vi "Set BME G05.vi"(7 "Settings":T1={"T Delay (µs)"=0.0, "T Set Back"=0.0, "T Triggers"=1, "T Active"=TRUE, "T Polarity"=TRUE, "T Term"=TRUE, "T Drive"=FALSE, "A Delay (µs)"=0.0, "A Set Back"=0.0, "A Triggers"=1, "A Active"=TRUE, "A Polarity"=TRUE, "A Term"=TRUE, "A Drive"=FALSE, "B Delay (µs)"=0.0, "B Set Back"=0.0, "B Triggers"=1, "B Active"=TRUE, "B Polarity"=TRUE, "B Term"=TRUE, "B Drive"=FALSE, "Gate A*B"=FALSE, "Output\nLevel"=1, "Trigger\nTerminate"=TRUE, "Clock\nEnable"=TRUE, "Internal\nClock (µs)"=0.0125, "Trigger\nLevel"=0.2, "Stop\nTrigger"=1, "Ocillator\nDivide By"=1, "Clock Source"=3, "Gate Divider"=1, "Positive\nGate"=FALSE, "Trigger\nSource"=FALSE, "Internal\nArming"=FALSE, "Software\nTrigger"=FALSE, "Trigger\nSlope"=TRUE, "Stop on\nPreset"=FALSE, "Trigger\nOperation"=TRUE, "Trigger\nEnable"=TRUE} {"B Set Back" min=0.0 format="%.3f"; "A Set Back" min=0.0 format="%.3f"; "T Set Back" min=0.0 format="%.3f"; "Clock Source" items=["Internal Oscillator"=1, "External Trigger"=2, "Trigger & Oscillator"=3, "Master Slave Bus"=4]; "Trigger\nLevel" min=0.0 format="%.3f"; "Output\nLevel" items=["TTL"=1, "NIM"=2, "ECL"=3]; "Internal\nClock (µs)" min=0.0 format="%.4f"; "B Delay (µs)" min=0.0 format="%.3f"; "A Delay (µs)" min=0.0 format="%.3f"; "T Delay (µs)" min=0.0 format="%.3f"}, 8 "error in (no error)":errorcluster, 10 "External Prescaler":u16=3, 11 "DG Number":i32) -> (0 "error out":errorcluster)   [LabVIEW 2009]
doc: "long Set_BME_G05(double FireFirst_T0, unsigned long OutputModulo_T0, BOOL Active_T0, BOOL Positive_T0, BOOL Terminate_T0, BOOL HighDrive_T0, double FireFirst_A, unsigned long OutputModulo_A, BOOL Active_A, BOOL Positive_A, BOOL Terminate_A, BOOL HighDrive_A, double FireFirst_B, unsigned long OutputModulo_B, BOOL Active_B, BOOL Positive_B, BOOL Terminate_B, BOOL HighDrive_B, BOOL Gate_AB, unsigned long OutputLevel, BOOL TriggerTerminate, BOOL ClockEnable, double InternalClock, double TriggerLevel, unsigned long PresetValue, unsigned long DivideBy, unsigned long ClockSource, unsigned long GateDivider, BOOL PositiveGate, BOOL InternalTrigger, BOOL InternalArm, BOOL SoftwareTrigger, BOOL RisingEdge, BOOL StopOnPreset, BOOL ResetWhenDone, BOOL TriggerEnable, long DG_Number);"
uses:
  Settings.ctl
  BME DLL/DelayGenerator.dll
panel:
  # "NOTICE -- YOU MUST LEAVE THIS NOTICE IN PLACE.  PER THE TERMS OF THE LICENSE BELOW, YOU MAY SUBLICENSE THIS SOFTWARE \nIN ANY WAY THAT DOES NOT CONFLICT WITH THIS LICENSE.\n\n### BSD License (http://www.opensource.org/licenses/bsd-license.php) Begin ###\n \nCopyright (c) 2011, Applied Energetics, http://www.appliedenergetics.com,\n                               Richard Schwerdtfeger, <rschwerdtfeger@appliedenergetics.com>\n\nAll rights reserved.\n\nRedistribution and use in source and binary forms, with or without modification, are permitted provided that the \nfollowing conditions are met:\n\n    * Redistributions of source code must retain the above copyright notice, this list of conditions and the following disclaimer.\n    * Redistributions in binary form must reproduce the above copyright notice, this list of conditions and the following disclaimer \n       in the documentation and/or other materials provided with the distribution.\n    * Neither the name of Richard Schwerdtfeger, Applied Energetics, Inc., nor the names of its contributors may be used to \n       endorse or promote products derived from this software without specific prior written permission.\n\nTHIS SOFTWARE IS PROVIDED BY THE COPYRIGHT HOLDERS AND CONTRIBUTORS \"AS IS\" AND ANY EXPRESS OR IMPLIED WARRANTIES, \nINCLUDING, BUT NOT LIMITED TO, THE IMPLIED WARRANTIES OF MERCHANTABILITY AND FITNESS FOR A PARTICULAR PURPOSE ARE \nDISCLAIMED. IN NO EVENT SHALL THE COPYRIGHT OWNER OR CONTRIBUTORS BE LIABLE FOR ANY DIRECT, INDIRECT, INCIDENTAL,\n SPECIAL, EXEMPLARY, OR CONSEQUENTIAL DAMAGES (INCLUDING, BUT NOT LIMITED TO, PROCUREMENT OF SUBSTITUTE GOODS OR \nSERVICES; LOSS OF USE, DATA, OR PROFITS; OR BUSINESS INTERRUPTION) HOWEVER CAUSED AND ON ANY THEORY OF LIABILITY, \nWHETHER IN CONTRACT, STRICT LIABILITY, OR TORT (INCLUDING NEGLIGENCE OR OTHERWISE) ARISING IN ANY WAY OUT OF THE USE \nOF THIS SOFTWARE, EVEN IF ADVISED OF THE POSSIBILITY OF SUCH DAMAGE.\n\n### BSD License End ###"
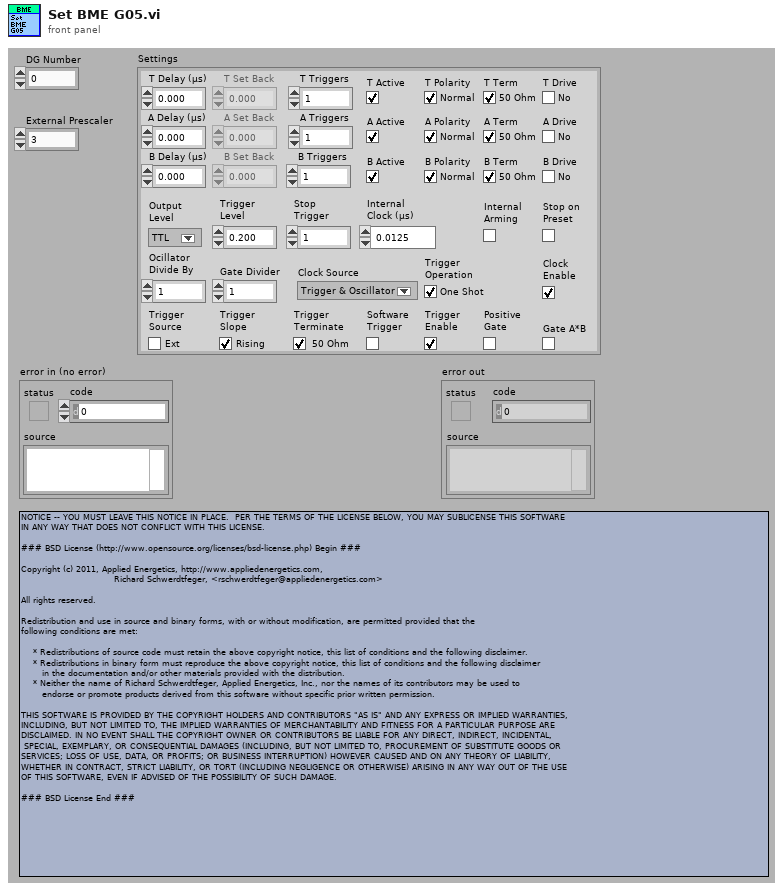
[diagram p1: front panel]
types:
  T1 = typedef "Settings.ctl" = cluster{"T Delay (µs)":dbl, "T Set Back":dbl, "T Triggers":u16, "T Active":bool, "T Polarity":bool, "T Term":bool, "T Drive":bool, "A Delay (µs)":dbl, "A Set Back":dbl, "A Triggers":u16, "A Active":bool, "A Polarity":bool, "A Term":bool, "A Drive":bool, "B Delay (µs)":dbl, "B Set Back":dbl, "B Triggers":u16, "B Active":bool, "B Polarity":bool, "B Term":bool, "B Drive":bool, "Gate A*B":bool, "Output\nLevel":u32, "Trigger\nTerminate":bool, "Clock\nEnable":bool, "Internal\nClock (µs)":dbl, "Trigger\nLevel":dbl, "Stop\nTrigger":u32, "Ocillator\nDivide By":u16, "Clock Source":u32, "Gate Divider":u32, "Positive\nGate":bool, "Trigger\nSource":bool, "Internal\nArming":bool, "Software\nTrigger":bool, "Trigger\nSlope":bool, "Stop on\nPreset":bool, "Trigger\nOperation":bool, "Trigger\nEnable":bool}
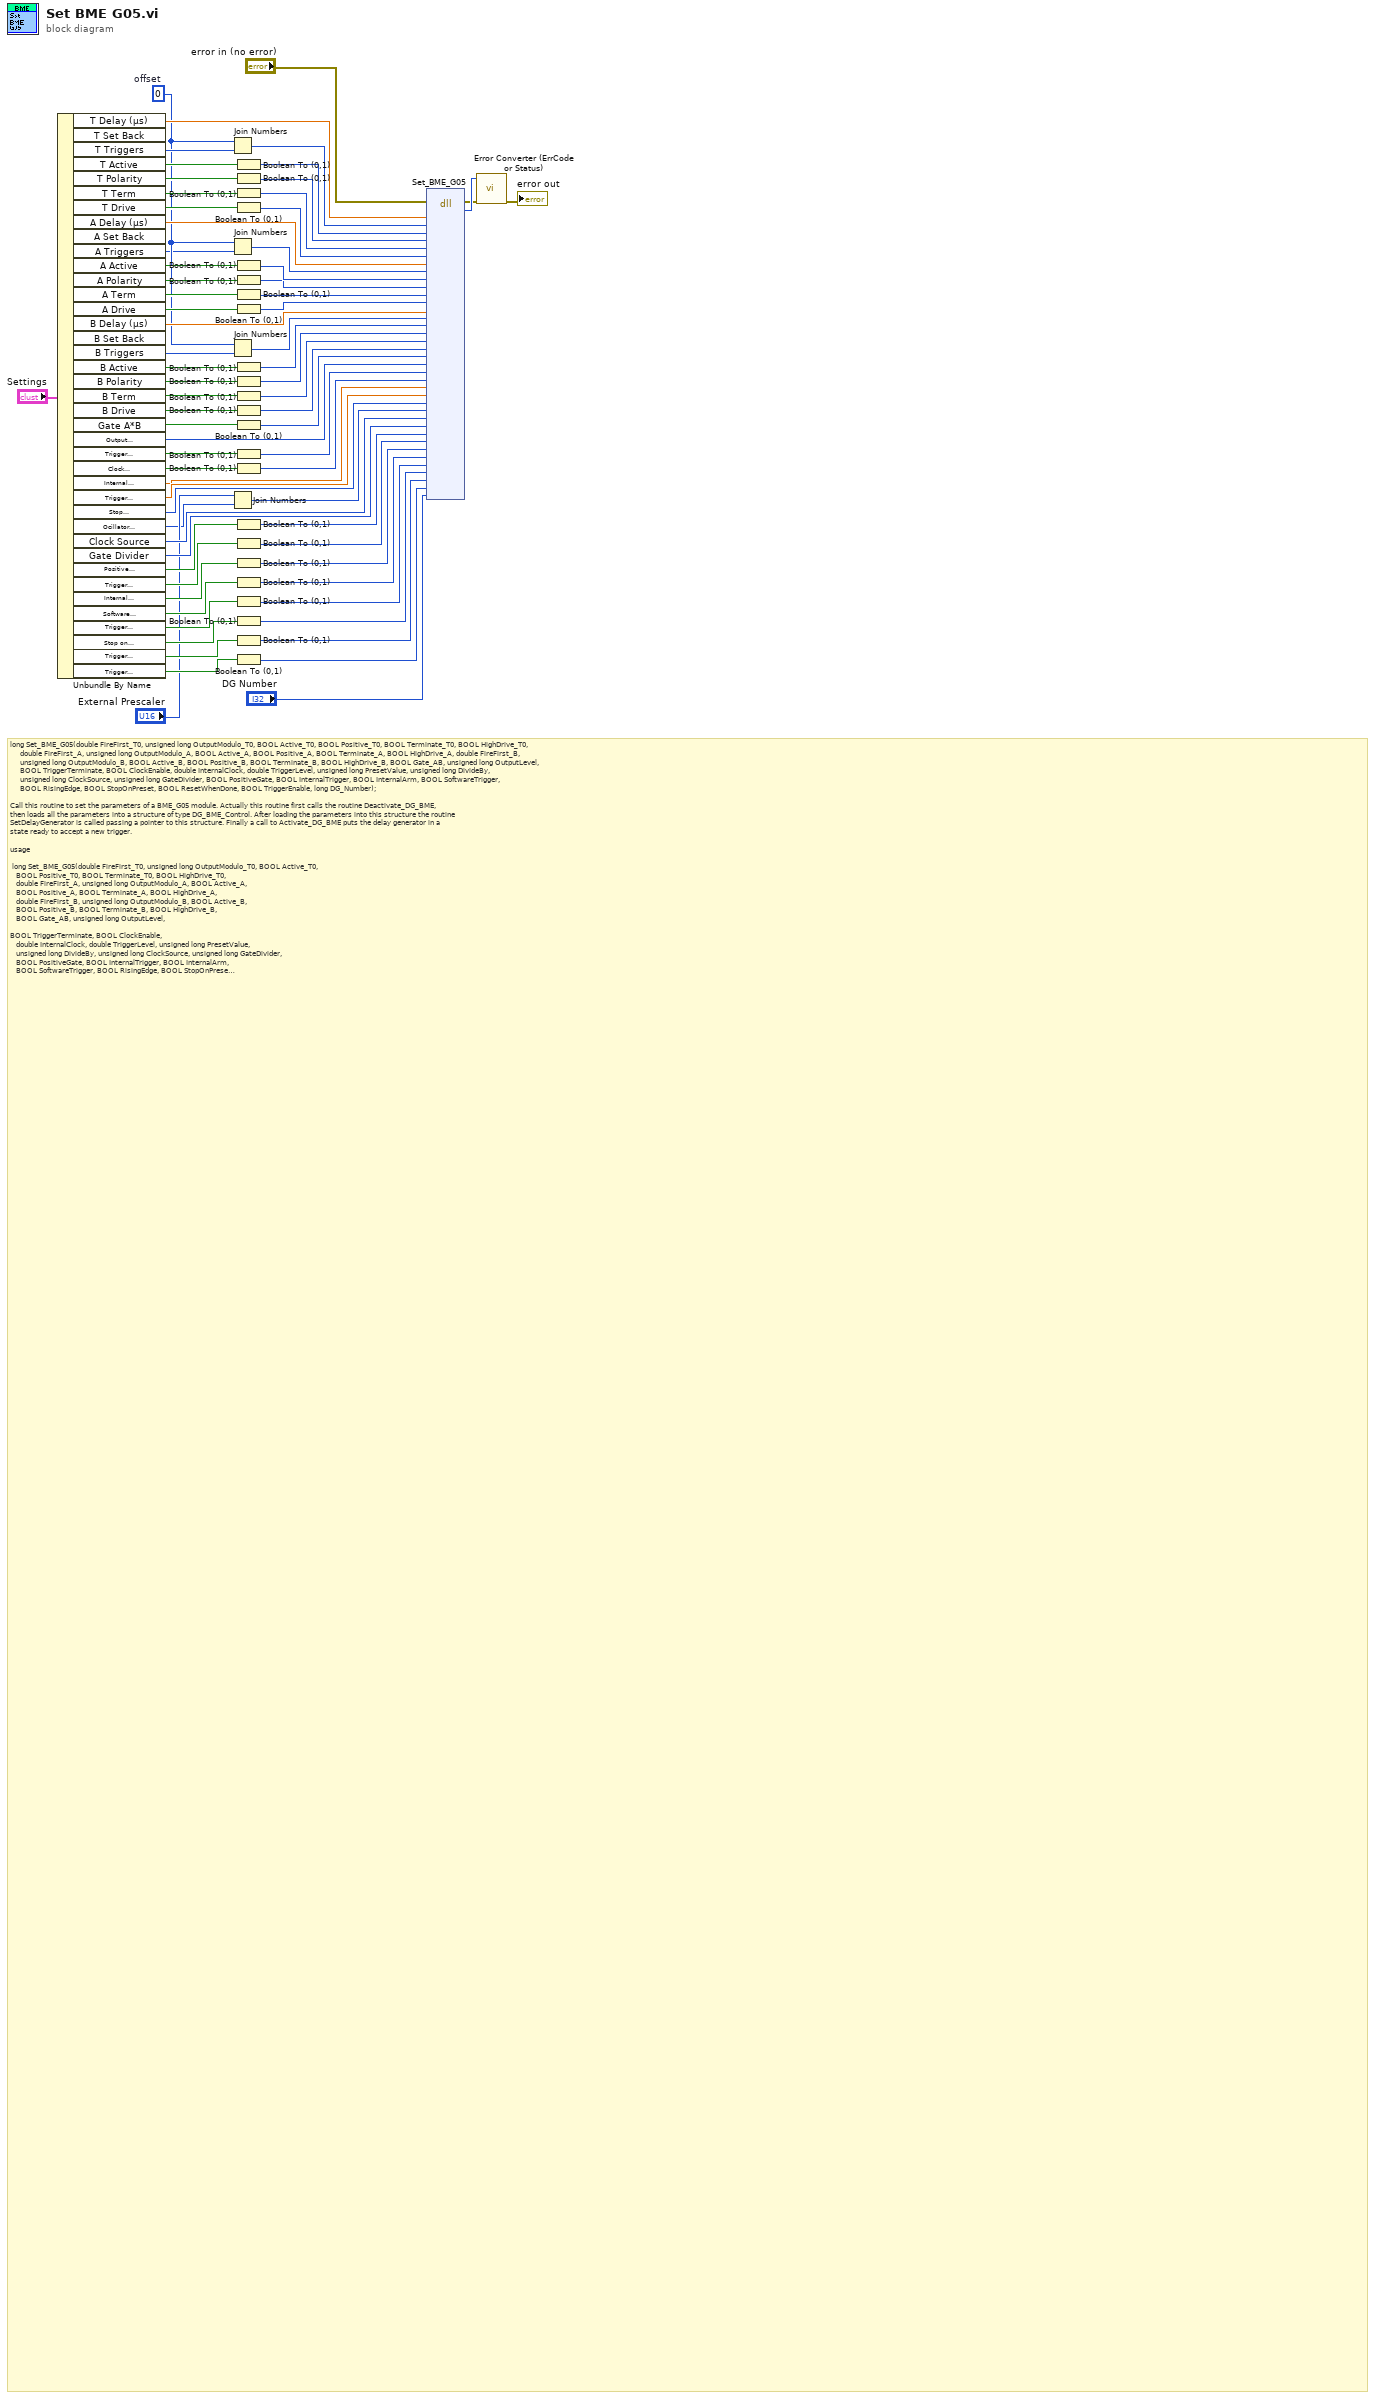
[diagram p0: block diagram]
diagram:
  w5 = u16 0  # offset
  # "long Set_BME_G05(double FireFirst_T0, unsigned long OutputModulo_T0, BOOL Active_T0, BOOL Positive_T0, BOOL Terminate_T0, BOOL HighDrive_T0, \n     double FireFirst_A, unsigned long OutputModulo_A, BOOL Active_A, BOOL Positive_A, BOOL Terminate_A, BOOL HighDrive_A, double FireFirst_B, \n     unsigned long OutputModulo_B, BOOL Active_B, BOOL Positive_B, BOOL Terminate_B, BOOL HighDrive_B, BOOL Gate_AB, unsigned long OutputLevel, \n     BOOL TriggerTerminate, BOOL ClockEnable, double InternalClock, double TriggerLevel, unsigned long PresetValue, unsigned long DivideBy, \n     unsigned long ClockSource, unsigned long GateDivider, BOOL PositiveGate, BOOL InternalTrigger, BOOL InternalArm, BOOL SoftwareTrigger, \n     BOOL RisingEdge, BOOL StopOnPreset, BOOL ResetWhenDone, BOOL TriggerEnable, long DG_Number);\n\nCall this routine to set the parameters of a BME_G05 module. Actually this routine first calls the routine Deactivate_DG_BME, \nthen loads all the parameters into a structure of type DG_BME_Control. After loading the parameters into this structure the routine \nSetDelayGenerator is called passing a pointer to this structure. Finally a call to Activate_DG_BME puts the delay generator in a \nstate ready to accept a new trigger.\n\nusage\n\n\tlong Set_BME_G05(double FireFirst_T0, unsigned long OutputModulo_T0, BOOL Active_T0,\n\t\t\tBOOL Positive_T0, BOOL Terminate_T0, BOOL HighDrive_T0,\n\t\t\tdouble FireFirst_A, unsigned long OutputModulo_A, BOOL Active_A,\n\t\t\tBOOL Positive_A, BOOL Terminate_A, BOOL HighDrive_A,\n\t\t\tdouble FireFirst_B, unsigned long OutputModulo_B, BOOL Active_B,\n\t\t\tBOOL Positive_B, BOOL Terminate_B, BOOL HighDrive_B,\n\t\t\tBOOL Gate_AB, unsigned long OutputLevel,\n\nBOOL TriggerTerminate, BOOL ClockEnable,\n\t\t\tdouble InternalClock, double TriggerLevel, unsigned long PresetValue,\n\t\t\tunsigned long DivideBy, unsigned long ClockSource, unsigned long GateDivider,\n\t\t\tBOOL PositiveGate, BOOL InternalTrigger, BOOL InternalArm,\n\t\t\tBOOL SoftwareTrigger, BOOL RisingEdge, BOOL StopOnPreset,\n\t\t\tBOOL ResetWhenDone, BOOL TriggerEnable, long DG_Number);\n\nparameters\n\nFireFirst_T0:    time after the main trigger in µsec, when the output T0 should be set\nOutputModulo_T0:    for every number of trigger events specified in this variable, only one pulse will actually be output at the T0 connector of the delay generator. \n\t\t\tActually this variable consists of two 16-bit numbers, the lower 16 bits actually specifying the number of triggers that have to occur for one pulse to come from the output connector. \n\t\t\tFor the delay generator models BME_G05P2 and BME_SG05P1 the higher 16 bits of this variable specify the offset when starting to count the triggers until a pulse comes from the \n\t\t\toutput connector. Note that after modifying this value, it is advisable to call the routine ResetOutputModuloCounters to resynchronize the output modulo counters.\nActive_T0:    TRUE to specify an output from T0, otherwise FALSE\nPositive_T0:    TRUE to specify a positive output polarity from T0, otherwise FALSE\nTerminate_T0:    TRUE to specify an internal 50 ohm termination on output T0, otherwise FALSE\nHighDrive_T0:    TRUE to specify a high current source driving a 25 ohm output, otherwise FALSE\n\nFireFirst_A:    time after the main trigger in µsec, when the output A should be set\nOutputModulo_A:    same as OutputModulo_T0 for output A\nActive_A:    TRUE to specify an output from A, otherwise FALSE\nPositive_A:    TRUE to specify a positive output polarity from A, otherwise FALSE\nTerminate_A:    TRUE to specify an internal 50 ohm termination on output A, otherwise FALSE\nHighDrive_A:    TRUE to specify a high current source driving a 25 ohm output, otherwise FALSE\n\nFireFirst_B:    time after the main trigger in µsec, when the output B should be set\nOutputModulo_B:    same as OutputModulo_T0 for output B\nActive_B:    TRUE to specify an output from B, otherwise FALSE\nPositive_B:    TRUE to specify a positive output polarity from B, otherwise FALSE\nTerminate_B:    TRUE to specify an internal 50 ohm termination on output B, otherwise FALSE\nHighDrive_B:    TRUE to specify a high current source driving a 25 ohm output, otherwise FALSE\n\nGate_AB:    if this flag is set, outputs A and B will be combined to form a gate signal, i.e. FireFirst_A will define the time when the output signal is set, and FireFirst_B will define the\n\t\t\ttime when the output signal is reset. Note that both outputs A and B must be activated, if the gate function is to be activated.\nOutputLevel:    specifies the voltage levels on the outputs of the delay generator. The constants for this variable are defined in ‘’DG_Data.h’’. (TTL_VoltageLevel, NIM_VoltageLevel, ECL_VoltageLevel)\nTriggerTerminate:    TRUE to specify an internal 50 ohm termination on the trigger input, otherwise FALSE\nClockEnable:    this flag must be set to enable the clock circuit\nInternalClock:    period of the internal clock in µsec. The BME_SG02p3 delay generator understands this entry as the trigger inhibit time.\nTriggerLevel:    Voltage of the trigger threshold. Can be varied from -2.5V to +2.5V\nPresetValue:    the BME_G02 will disable its trigger circuit after this number of trigger signals has occurred, provided the StopOnPreset flag is set.\nDivideBy:    this variable consists of two 16-bit unsigned short values. The lower signifying the prescaler value of the internal quarz oscillator, the higher giving the prescaler value for the \n\t\t\texternal clock signal fed via the trigger input connector\nClockSource:        the source of the clock signal, can be the crystal oscillator or a signal fed to the external trigger input. (The constants for this variable, CrystalOscillator or TriggerInput, are defined in ‘’DG_Data.h’’.)\n    CrystalOscillator = 1:    internal quarz oscillator is used\n    TriggerInput = 2:         signal from external trigger/clock input connector is used\n    TriggerAndOscillator = 3:     like TriggerInput, but if this signal fails, the signal from the internal quarz oscillator will be used.\n\nGateDivider:    the external gate signal will be divided by this number.\nPositiveGate:    set this flag to TRUE, if a positive signal on the external gate input should enable the trigger circuit, otherwise FALSE. Note that the TriggerEnable flag is or’ed \n\t\t\twith the external gate signal. Only when the TriggerEnable flag is set FALSE, the trigger circuit can be enabled by the external gate signal.\nInternalTrigger:    if this flag is set the BME_G02 will be triggered by its internal clock, (provided it is jumpered as a master module).\nInternalArm:    if this flag is set the external trigger of the BME_G02 will be armed by its internal clock, (provided it is jumpered as a master module).\nSoftwareTrigger:        if this flag is set the BME_G02 will be triggered by the SoftwareTrigger_DG_BME routine, (provided it is jumpered as a master module). The flags InternalTrigger and\n\t\t\t SoftwareTrigger may not be set at the same time.\nRisingEdge:    if none of the flags InternalTrigger or SoftwareTrigger are set and this module is jumpered as master, the BME_G02 will be triggered by the rising edge of a signal applied to its external connector.\nStopOnPreset:    if this flag is set, the BME_G02 will disable its trigger circuit when the number of triggers prescribed by PresetValue has been reached. Modules slaved to a master will also stop at this point.\nResetWhenDone:    if this flag is set, all outputs from master and slave(s) will be reset to their untriggered states 2 µsec after the last delay of master and slave(s) has elapsed. This function is controlled by \n\t\t\tthe master module. If this flag is not set, all modules, master and slave(s) have to be individually reset by calling the two routines Deactivate_DG_BME and Activate_DG_BME (in that order).\nTriggerEnable:    this flag must be set to enable the trigger circuit. This signal is or'ed with the signal coming from the external gate input. Actually, the rising edge of the (divided) gate signal clocks a flip-flop \n\t\t\tallowing a trigger. After a trigger has occurred, the flip-flop is reset.\nDG_Number:    The number of the delay generator as assigned by the Initialize_DG_BME routine\n\n\nreturn value\n\n0:  success\n2:  DG_Number is out of range\n3:  the FireFirst time of an output is negative while the Active flag is TRUE.\n4:  more than one of the flags InternalTrigger, InternalArm, and SoftwareTrigger have both been set\n5:  one or more delay time(s) is specified too long\n6:  parameter ‘OutputLevel’ has been passed with illegal value. (See DG_Data.h)\n7:  parameter ‘ClockSource’ has been passed with illegal value. (See DG_Data.h)"
  n1 = Unbundle By Name("Settings") -> ("T Delay (µs)"=w44:dbl, "T Triggers"=w7:u16, "T Active"=w47:bool, "T Polarity"=w48:bool, "T Term"=w49:bool, "T Drive"=w50:bool, "A Delay (µs)"=w39:dbl, "A Triggers"=w2:u16, "A Active"=w51:bool, "A Polarity"=w52:bool, "A Term"=w53:bool, "A Drive"=w54:bool, "B Delay (µs)"=w34:dbl, "B Triggers"=w1:u16, "B Active"=w58:bool, "B Polarity"=w55:bool, "B Term"=w56:bool, "B Drive"=w57:bool, "Gate A*B"=w61:bool, "Output\nLevel"=w28:u32, "Trigger\nTerminate"=w59:bool, "Clock\nEnable"=w60:bool, "Internal\nClock (µs)"=w8:dbl, "Trigger\nLevel"=w25:dbl, "Stop\nTrigger"=w24:u32, "Ocillator\nDivide By"=w10:u16, "Clock Source"=w13:u32, "Gate Divider"=w14:u32, "Positive\nGate"=w62:bool, "Trigger\nSource"=w12:bool, "Internal\nArming"=w63:bool, "Software\nTrigger"=w64:bool, "Trigger\nSlope"=w65:bool, "Stop on\nPreset"=w66:bool, "Trigger\nOperation"=w67:bool, "Trigger\nEnable"=w68:bool)  [unwired: 3 out]
  n2 = Join Numbers(hi=w5, lo=w7) -> ((hi.lo)=w6:u32)
  n3 = Join Numbers(hi=w5, lo=w2) -> ((hi.lo)=w4:u32)
  n4 = Join Numbers(hi=w5, lo=w1) -> ((hi.lo)=w3:u32)
  n5 = Join Numbers(hi="External Prescaler", lo=w10) -> ((hi.lo)=w9:u32)
  n6 = Boolean To (0,1)(Boolean=w47) -> (0, 1=w43:i16)
  n7 = Boolean To (0,1)(Boolean=w48) -> (0, 1=w42:i16)
  n8 = Boolean To (0,1)(Boolean=w49) -> (0, 1=w41:i16)
  n9 = Boolean To (0,1)(Boolean=w50) -> (0, 1=w40:i16)
  n10 = Boolean To (0,1)(Boolean=w51) -> (0, 1=w38:i16)
  n11 = Boolean To (0,1)(Boolean=w52) -> (0, 1=w37:i16)
  n12 = Boolean To (0,1)(Boolean=w53) -> (0, 1=w36:i16)
  n13 = Boolean To (0,1)(Boolean=w54) -> (0, 1=w35:i16)
  n14 = Boolean To (0,1)(Boolean=w58) -> (0, 1=w33:i16)
  n15 = Boolean To (0,1)(Boolean=w55) -> (0, 1=w32:i16)
  n16 = Boolean To (0,1)(Boolean=w56) -> (0, 1=w31:i16)
  n17 = Boolean To (0,1)(Boolean=w57) -> (0, 1=w30:i16)
  n18 = Boolean To (0,1)(Boolean=w61) -> (0, 1=w29:i16)
  n19 = Boolean To (0,1)(Boolean=w59) -> (0, 1=w27:i16)
  n20 = Boolean To (0,1)(Boolean=w60) -> (0, 1=w26:i16)
  n21 = Boolean To (0,1)(Boolean=w62) -> (0, 1=w15:i16)
  n22 = Boolean To (0,1)(Boolean=w12) -> (0, 1=w16:i16)
  n23 = Boolean To (0,1)(Boolean=w63) -> (0, 1=w17:i16)
  n24 = Boolean To (0,1)(Boolean=w64) -> (0, 1=w18:i16)
  n25 = Boolean To (0,1)(Boolean=w65) -> (0, 1=w19:i16)
  n26 = Boolean To (0,1)(Boolean=w66) -> (0, 1=w20:i16)
  n27 = Boolean To (0,1)(Boolean=w67) -> (0, 1=w21:i16)
  n28 = Boolean To (0,1)(Boolean=w68) -> (0, 1=w22:i16)
  n29 = dll-call lib="C:/Dokumente und Einstellungen/A2.5/Desktop/POLARIS BME DG/BME DLL/DelayGenerator.*" fn="Set_BME_G05"(error in="error in (no error)", "FireFirst_T0"=w44, "OutputModulo_T0"=w6, "Active_T0"=w43, "Positive_T0"=w42, "Terminate_T0"=w41, "HighDrive_T0"=w40, "FireFirst_A"=w39, "OutputModulo_A"=w4, "Active_A"=w38, "Positive_A"=w37, "Terminate_A"=w36, "HighDrive_A"=w35, "FireFirst_B"=w34, "OutputModulo_B"=w3, "Active_B"=w33, "Positive_B"=w32, "Terminate_B"=w31, "HighDrive_B"=w30, "Gate_AB"=w29, "OutputLevel"=w28, "TriggerTerminate"=w27, "ClockEnable"=w26, "InternalClock"=w8, "TriggerLevel"=w25, "PresetValue"=w24, "DivideBy"=w9, "ClockSource"=w13, "GateDivider"=w14, "PositiveGate"=w15, "InternalTrigger"=w16, "InternalArm"=w17, "SoftwareTrigger"=w18, "RisingEdge"=w19, "StopOnPreset"=w20, "ResetWhenDone"=w21, "TriggerEnable"=w22, "DG_Number"="DG Number") -> (error out=w70:errorcluster, "return type"=w71:i32)  [unwired: 39 in, 1 out]
  n30 = call "Error Converter (ErrCode or Status).vi"("error in (no error)"=w70, "error code"=w71) -> ("error out"=→"error out":errorcluster)  [unwired: 9 out]
